vi "MListbox Initialize Cell.vi"(8 "error in (no error)":errorcluster, 10 "Initialize":cluster{"Row":u16, "Colunm":u16}, 11 "Multicolumn ListBox in":refnum<class "Multicolumn ListBox.lvclass">) -> (0 "error out":errorcluster, 3 "Multicolumn ListBox out":refnum<class "Multicolumn ListBox.lvclass">)   [LabVIEW 2012, in "Multicolumn ListBox.lvclass"]
uses:
  Multicolumn ListBox.lvclass
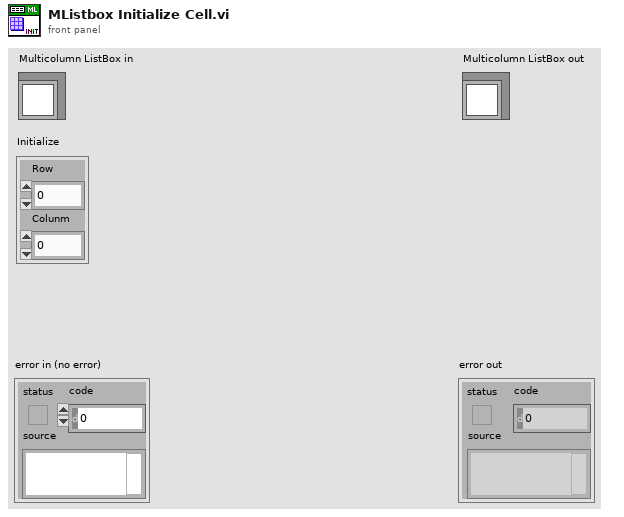
[diagram p1: front panel]
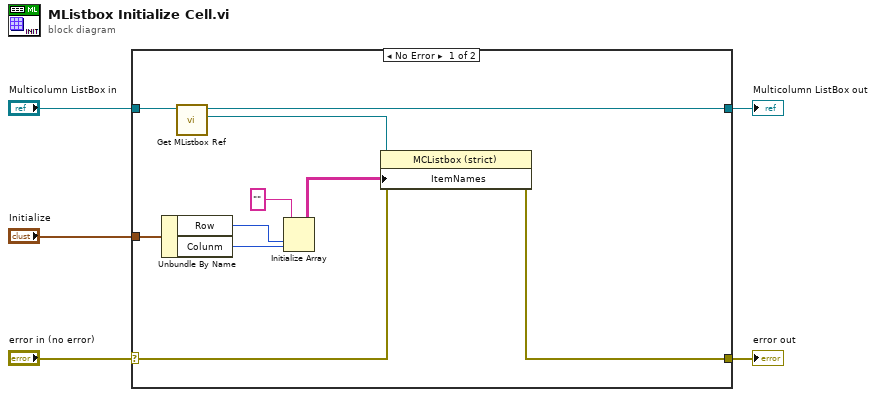
[diagram p0: block diagram]
diagram:
  n1 = case shown="No Error" "error in (no error)" {
    selector: "error in (no error)" -> [w11 w17]
    tunnel: [w6 w17] -> w4
    tunnel: [w14 w16] -> w2
    tunnel: "Multicolumn ListBox in" -> [w15 w16]
    tunnel: "Initialize" -> [w12 _]
    frame No Error {
      n2 = Unbundle By Name(w12) -> ("Row"=w10:u16, "Colunm"=w9:u16)
      n3 = call "Get MListbox Ref.vi"("Multicolumn ListBox in"=w15) -> ("MListbox Ref"=w13:refnum<vi>, "Multicolumn ListBox out"=w14:refnum<class "Multicolumn ListBox.lvclass">)  [unwired: 8 in, 1 out]
      n4 = Initialize Array("", w10, w9) -> (w7:string[][])
      n5 = property class="MCListbox (strict)"(reference=w13, error in=w11, "ItemNames"=w7) -> (error out=w6:errorcluster)  [unwired: 1 out]
    }
    frame Error {
    }
  }
  "error out" <- w4
  "Multicolumn ListBox out" <- w2
